vi "LR700_ReadDeltaRandR0.vi"(8 "error in (no error)":errorcluster, 11 "LR700\nAddress":i16) -> (0 "error out":errorcluster, 2 "R0":dbl, 3 "DeltaR":dbl)   [LabVIEW 2014]
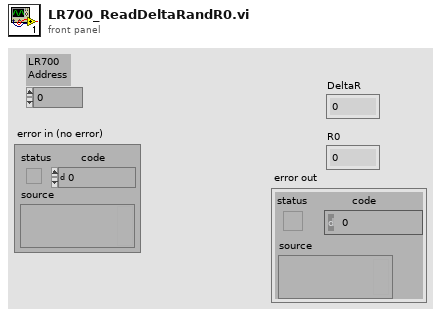
[diagram p1: front panel]
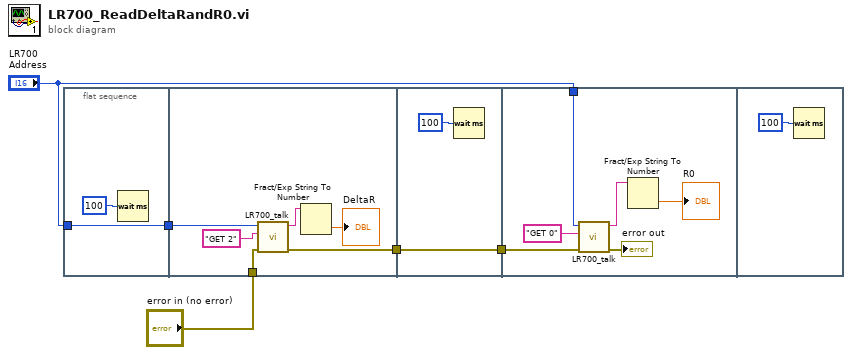
[diagram p0: block diagram]
diagram:
  n1 = flat-sequence {
    tunnel: "LR700\nAddress" -> [w7]
    tunnel: [w7] -> w1
    tunnel: "error in (no error)" -> [w10]
    tunnel: [w8] -> w3
    tunnel: w1 -> [w11]
    tunnel: w3 -> [w15]
    tunnel: [w15] -> w2
    tunnel: "LR700\nAddress" -> [w17]
    tunnel: w2 -> [w16]
    frame #0 {
      n2 = Wait (ms)(milliseconds to wait=100) -> ()  [unwired: 1 out]
    }
    frame #1 {
      n3 = call "LR700_talk.vi"("error in"=w10, "Send"="GET 2", "Address"=w11) -> ("error out"=w8:errorcluster, "read"=w13:string)  [unwired: 7 in]
      n4 = Fract/Exp String To Number(string=w13) -> (number=→"DeltaR":dbl)  [unwired: 3 in, 1 out]
    }
    frame #2 {
      n5 = Wait (ms)(milliseconds to wait=100) -> ()  [unwired: 1 out]
    }
    frame #3 {
      n6 = call "LR700_talk.vi"("error in"=w16, "Send"="GET 0", "Address"=w17) -> ("error out"=→"error out":errorcluster, "read"=w20:string)  [unwired: 7 in]
      n7 = Fract/Exp String To Number(string=w20) -> (number=→"R0":dbl)  [unwired: 3 in, 1 out]
    }
    frame #4 {
      n8 = Wait (ms)(milliseconds to wait=100) -> ()  [unwired: 1 out]
    }
  }
